vi "罗列文件.vi"() -> ()   [LabVIEW 2018]
panel:
  out "文件名输出":string[](array[string])
  in  "模式":string
  out "路径输出":path
  in  "路径":path
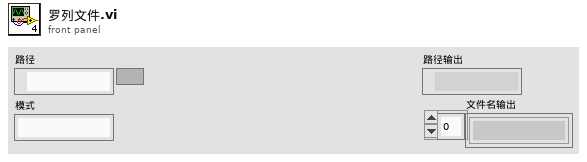
[diagram p1: front panel]
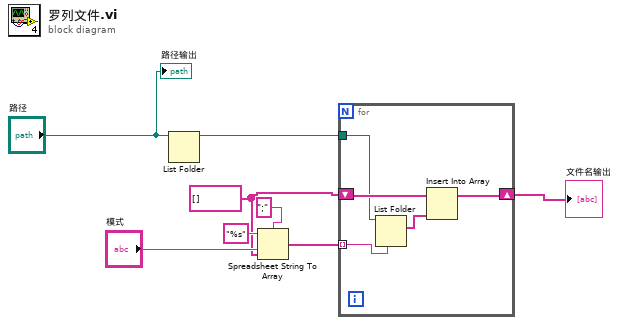
[diagram p0: block diagram]
diagram:
  w4 = string[] []
  n1 = List Folder(path="路径") -> (path out=w1:path)  [unwired: 3 in, 3 out]
  n2 = Spreadsheet String To Array(delimiter (Tab)=";", format string="%s" ("格式字符串"), spreadsheet string="模式", array type (2D Dbl)=w4) -> (array=w3:string[])
  n3 = for {
    shift-right: [w12] -> w2
    shift-left: w4 -> [w13]
    tunnel: w3 -> [w11] mode=indexing
    tunnel: w1 -> [w9]
    n4 = List Folder(path=w9, pattern=w11) -> (filenames=w10:string[])  [unwired: 2 in, 3 out]
    n5 = Insert Into Array(array=w13, new element=w10) -> (w12:string[])  [unwired: 1 in]
  }
  "文件名输出" <- w2
  "路径输出" <- "路径"
